vi "Lift Teleop Call.vi"(9 "POVs":i16[](array[numeric]), 10 "Button Values":bool[](array[boolean])) -> ()   [LabVIEW 2017]
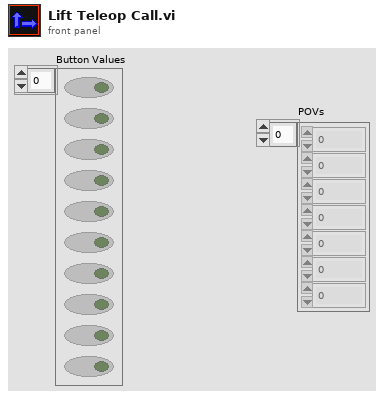
[diagram p1: front panel]
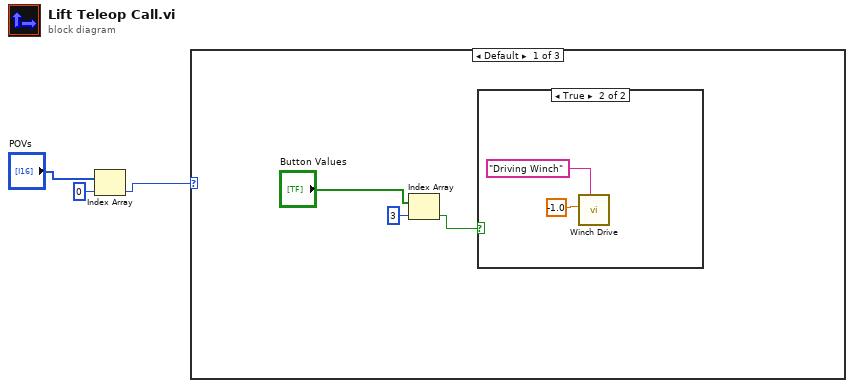
[diagram p0: block diagram]
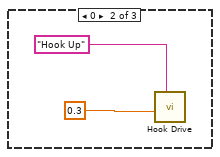
[diagram p3: hidden frame]
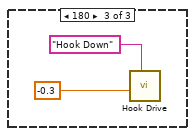
[diagram p4: hidden frame]
diagram:
  n1 = Index Array(array="POVs", index=0) -> (element=w1:i16)
  n2 = case shown="Default" w1 {
    frame Default {
      n3 = Index Array(array="Button Values", index=3) -> (element=w5:bool)
      n4 = case shown="True" w5 {
        frame False {
        }
        frame True {
          n5 = call "Winch Drive.vi"("Description"="Driving Winch", "Winch Motor"=-1.0) -> ()  [unwired: 9 in, 1 out]
        }
      }
    }
    frame 0 {
      n6 = call "Hook Drive.vi"("Description"="Hook Up", "Hook Motor"=0.3) -> ()  [unwired: 9 in, 1 out]
    }
    frame 180 {
      n7 = call "Hook Drive.vi"("Description"="Hook Down", "Hook Motor"=-0.3) -> ()  [unwired: 9 in, 1 out]
    }
  }
